vi "Read Pane Dimension.vi"(9 "Tab in":refnum<class "Tab.lvclass">) -> (3 "Tab out":refnum<class "Tab.lvclass">, 4 "Pane Dimension":T1)   [LabVIEW 2014, in "Raspberry Pi Compatible Compiler for LabVIEW.lvlib" / "Tab.lvclass"]
uses:
  Tab.lvclass
  <vilib>/Utility/miscctls.llb/LVPointTypeDef.ctl
  Tab.lvclass/Tab.ctl
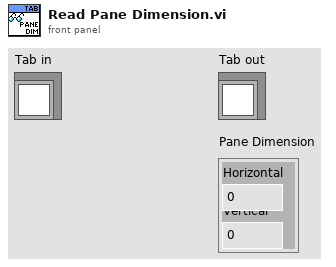
[diagram p1: front panel]
types:
  T1 = typedef "LVPointTypeDef.ctl" = cluster{"Horizontal":i16, "Vertical":i16}
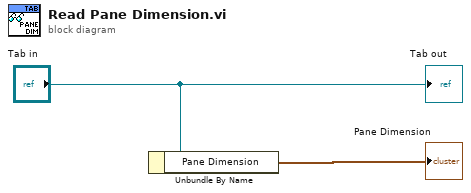
[diagram p0: block diagram]
diagram:
  n1 = Unbundle By Name("Tab in") -> ("Pane Dimension"=→"Pane Dimension":T1)
  "Tab out" <- "Tab in"
